vi "Operations.vi"(7 "References":T2, 8 "error in":errorcluster, 9 "BD":T1 items=["Server", "Local DB"], 10 "FilesPath":path, 11 "Queues in":T9) -> (0 "error out":errorcluster, 2 "Prop out":T12={"Raw Data"=[[0.0], [0.0234375], [0.9609375]], "Poperties"={"RMS values"=[], "Max"=[], "Min"=[], "A(8)"=[], "t"=0.0, "A(8) Axis"=0.0, "Aw"=[], "Ak 30min"=0.0, "Ak_axis"=0, "Spec"=[]}, "Power Spectrum / PSD"=[]}, 3 "Queues out":T9)   [LabVIEW 2019]
uses:
  Communication/TypeDef/#TypeDef_PropGraph.ctl
  Communication/TypeDef/#TypeDef_PropertiesToSave.ctl
  Queue/TypeDef/#TypeDef_App_Queues.ctl
  User Interface/TypeDef/#TypeDef_Enum_Buttons.ctl
  User Interface/TypeDef/#TypeDef_EventStructureConstant.ctl
  User Interface/TypeDef/#TypeDef_Enum_EventStructure.ctl
  Queue/TypeDef/#TypeDef_NetworkStream.ctl
  Communication/TypeDef/#TypeDef_FromMRtoPC.ctl
  Communication/TypeDef/#TypeDef_FromPCtoMR.ctl
  Communication/TypeDef/#TypeDef_Command.ctl
  Communication/TypeDef/#TypeDef_ErrorHandler_prop.ctl
  <vilib>/addons/database/Connection.llb/Conn ObjectReference.ctl
  Test/TypeDef/#TypeDef_DataToTest.ctl
  User Interface/TypeDef/#TypeDef_References.ctl
  User Interface/TypeDef/#TypeDef_Buttons.ctl
  User Interface/TypeDef/#TypeDef_ReferencesMeassurementProp.ctl
  User Interface/TypeDef/#TypeDef_ReferencesArchiveProp.ctl
  User Interface/TypeDef/#TypeDef_Lists.ctl
  User Interface/TypeDef/#TypeDef_MeasProp.ctl
  User Interface/TypeDef/#TypeDef_OpProp.ctl
  User Interface/TypeDef/#TypeDef_Enum_ModeOp.ctl
  DataBase/TypeDef/#TypeDef_DBMode.ctl
  DataBase/TypeDef/#TypeDef_FinalDataToDatabase.ctl
  Communication/TypeDef/#TypeDef_SetGet.ctl
  <vilib>/addons/database/NI_Database_API.lvlib
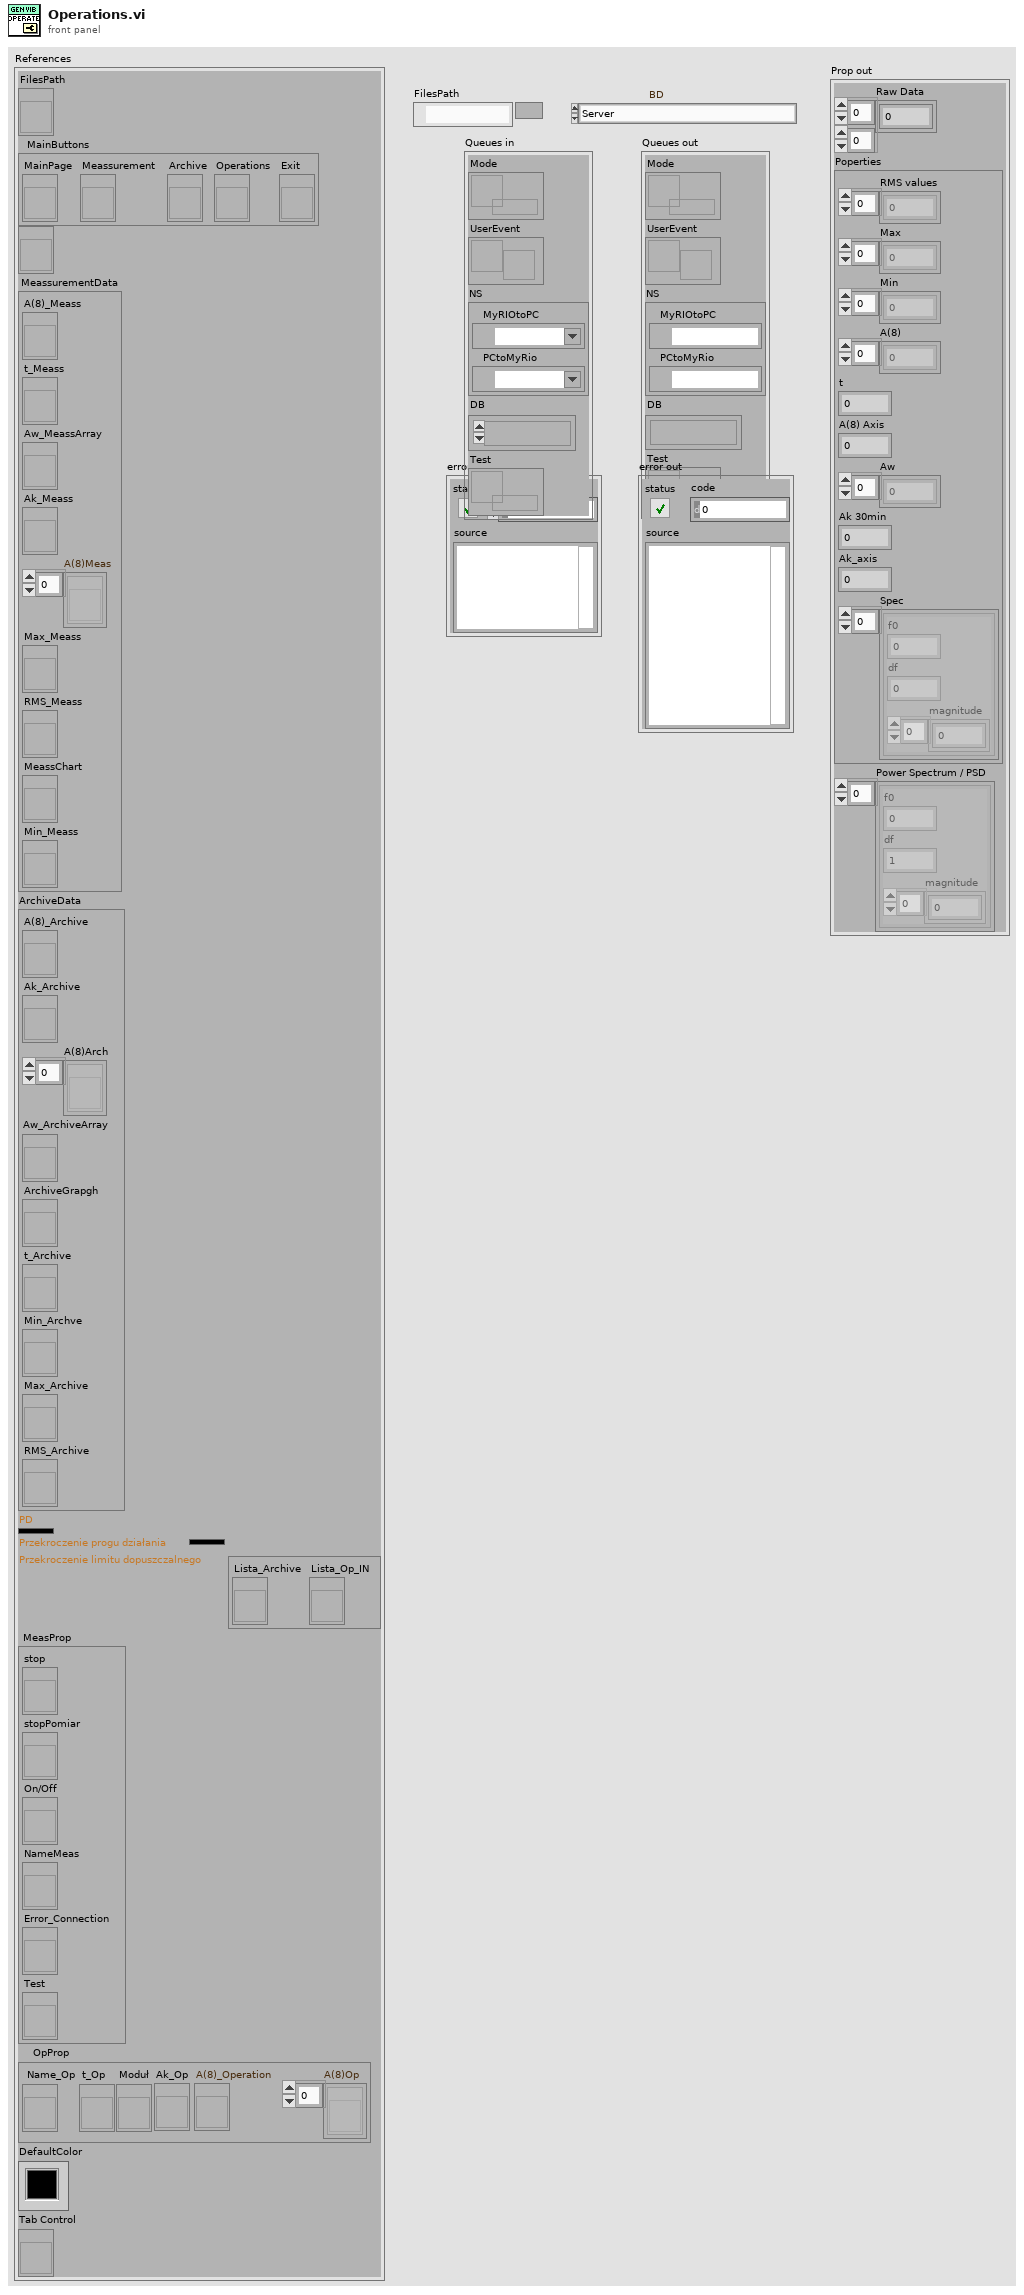
[diagram p1: front panel]
types:
  T1 = typedef "#TypeDef_DBMode.ctl" = u16
  T2 = typedef "#TypeDef_References.ctl" = cluster{"FilesPath":refnum<vi>, "MainButtons":T3, "Lista CTRL":refnum<vi>, "MeassurementData":T4, "ArchiveData":T5, "PD":u32, "LD":u32, "Lists":T6, "MeasProp":T7, "OpProp":T8, "DefaultColor":u32, "Tab Control":refnum<vi>}
  T3 = typedef "#TypeDef_Buttons.ctl" = cluster{"MainPage":refnum<vi>, "Meassurement":refnum<vi>, "Archive":refnum<vi>, "Operations":refnum<vi>, "Exit":refnum<vi>}
  T4 = typedef "#TypeDef_ReferencesMeassurementProp.ctl" = cluster{"A(8)_Meass":refnum<vi>, "t_Meass":refnum<vi>, "Aw_MeassArray":refnum<vi>, "Ak_Meass":refnum<vi>, "A(8)Meas":refnum<vi>[], "Max_Meass":refnum<vi>, "RMS_Meass":refnum<vi>, "MeassChart":refnum<vi>, "Min_Meass":refnum<vi>}
  T5 = typedef "#TypeDef_ReferencesArchiveProp.ctl" = cluster{"A(8)_Archive":refnum<vi>, "Ak_Archive":refnum<vi>, "A(8)Arch":refnum<vi>[], "Aw_ArchiveArray":refnum<vi>, "ArchiveGrapgh":refnum<vi>, "t_Archive":refnum<vi>, "Min_Archve":refnum<vi>, "Max_Archive":refnum<vi>, "RMS_Archive":refnum<vi>}
  T6 = typedef "#TypeDef_Lists.ctl" = cluster{"Lista_Archive":refnum<vi>, "Lista_Op_IN":refnum<vi>}
  T7 = typedef "#TypeDef_MeasProp.ctl" = cluster{"stop":refnum<vi>, "stopPomiar":refnum<vi>, "On/Off":refnum<vi>, "NameMeas":refnum<vi>, "Error_Connection":refnum<vi>, "Test":refnum<vi>}
  T8 = typedef "#TypeDef_OpProp.ctl" = cluster{"Name_Op":refnum<vi>, "t_Op":refnum<vi>, "Modu³":refnum<vi>, "Ak_Op":refnum<vi>, "A(8)_Operation":refnum<vi>, "A(8)Op":refnum<vi>[]}
  T9 = typedef "#TypeDef_App_Queues.ctl" = cluster{"Mode":refnum<queue>, "UserEvent":refnum<user-event>, "NS":T10, "DB":T11, "Test":refnum<queue>}
  T10 = typedef "#TypeDef_NetworkStream.ctl" = cluster{"MyRIOtoPC":refnum<k21>, "PCtoMyRio":refnum<k21>}
  T11 = typedef "NI_Database_API.lvlib/Conn ObjectReference.ctl" = refnum<k1>
  T12 = typedef "#TypeDef_PropGraph.ctl" = cluster{"Raw Data":dbl[][], "Poperties":T13, "Power Spectrum / PSD":cluster{"f0":dbl, "df":dbl, "magnitude":dbl[]}[]}
  T13 = typedef "#TypeDef_PropertiesToSave.ctl" = cluster{"RMS values":dbl[], "Max":dbl[], "Min":dbl[], "A(8)":dbl[], "t":dbl, "A(8) Axis":dbl, "Aw":dbl[], "Ak 30min":dbl, "Ak_axis":i32, "Spec":cluster{"f0":dbl, "df":dbl, "magnitude":dbl[]}[]}
  T14 = enum16{"open", "open or create", "create or replace", "create", "open (read-only)"}
  T15 = typedef "#TypeDef_SetGet.ctl" = enum16{"Set", "Get"}
  T16 = typedef "#TypeDef_FinalDataToDatabase.ctl" = cluster{"A8":dbl[], "Ak Aray":dbl[]}
  T17 = typedef "#TypeDef_Enum_ModeOp.ctl" = enum16{"Oblicz ekspozycjê dzienn¹", "Uœrednij"}
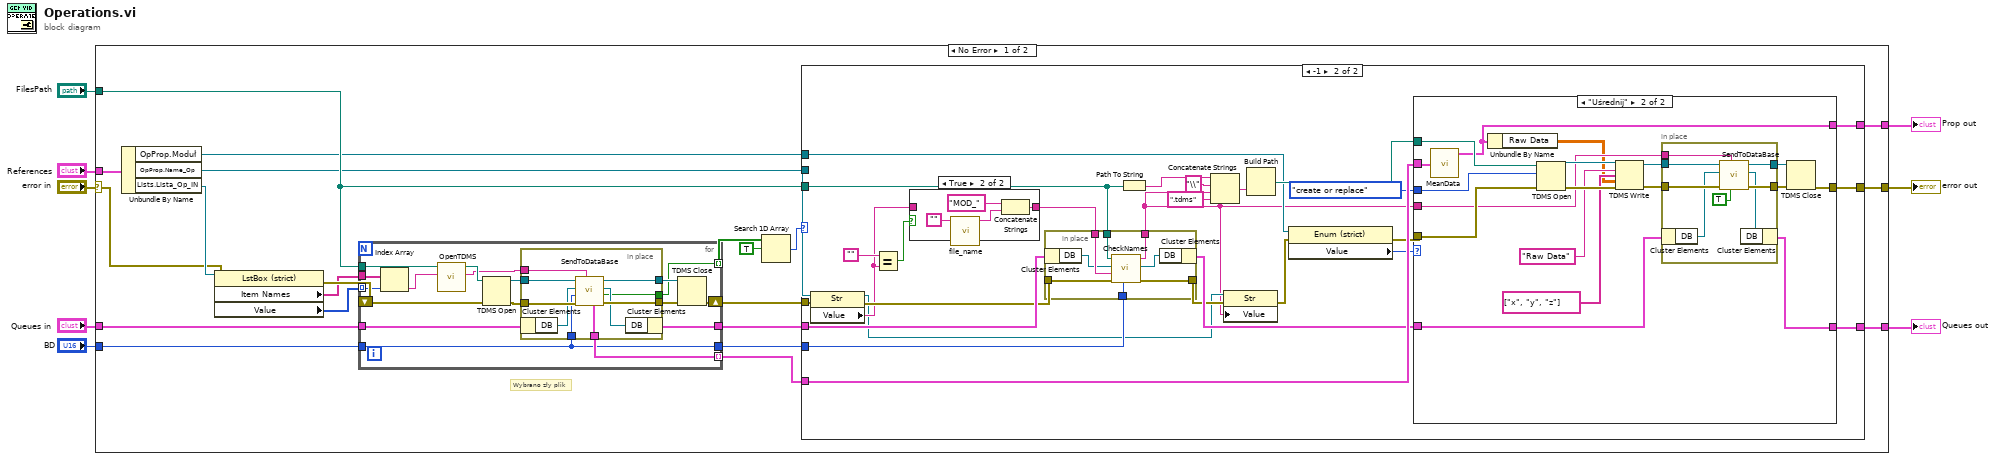
[diagram p0: block diagram]
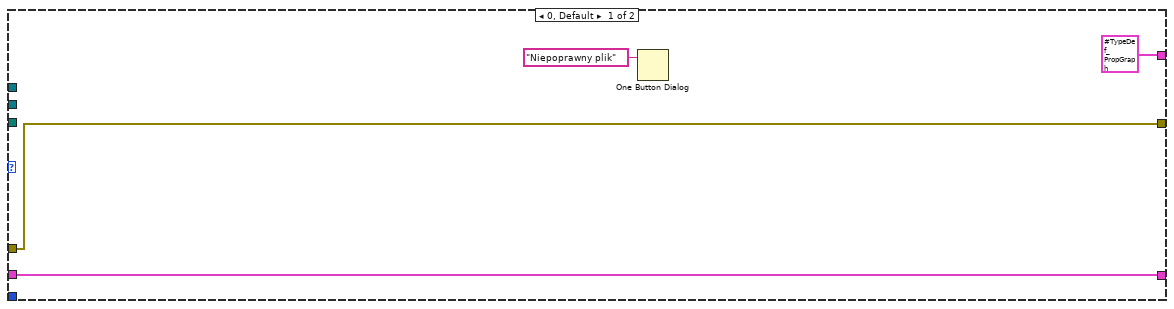
[diagram p2: hidden frame]
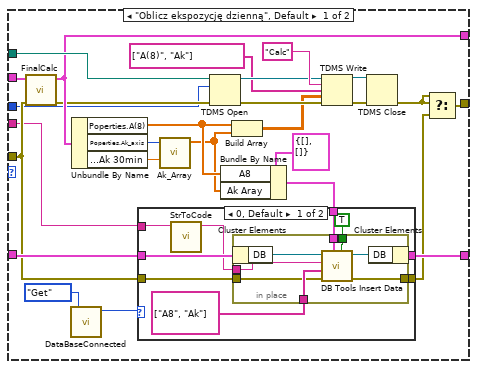
[diagram p4: hidden frame]
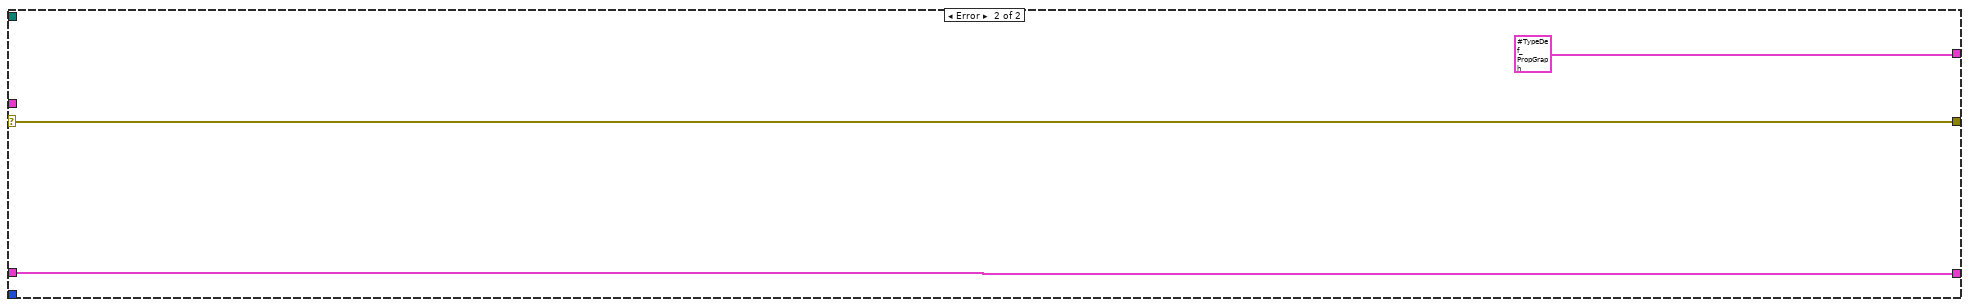
[diagram p6: hidden frame]
diagram:
  n1 = case shown="No Error" "error in" {
    selector: "error in" -> [w18 w174]
    tunnel: [w29 T12 {"Raw Data"=[[0.0], [0.0234375], [0.9609375]], "Poperties"={"RMS values"=[], "Max"=[], "Min"=[], "A(8)"=[], "t"=0.0, "A(8) Axis"=0.0, "Aw"=[], "Ak 30min"=0.0, "Ak_axis"=0, "Spec"=[]}, "Power Spectrum / PSD"=[]} ("Prop out")] -> w2
    tunnel: [w21 w175] -> w7
    tunnel: "Queues in" -> [w26 w175]
    tunnel: "References" -> [w24 _]
    tunnel: "FilesPath" -> [w22 _]
    tunnel: [w23 w174] -> w3
    tunnel: "BD" -> [w16 _]
    frame No Error {
      # "Wybrano z³y plik"
      n2 = Unbundle By Name(w24) -> ("OpProp.Modu³"=w17:refnum<vi>, "OpProp.Name_Op"=w12:refnum<vi>, "Lists.Lista_Op_IN"=w25:refnum<vi>)
      n3 = property class="LstBox (strict)"(reference=w25, error in=w18) -> (error out=w27:errorcluster, "Item Names"=w20:string[], "Value"=w19:i32[])  [unwired: 1 out]
      n4 = for {
        tunnel: w26 -> [w162]
        tunnel: [w161] -> w14
        shift-right: [w151] -> w13
        shift-left: w27 -> [w160]
        tunnel: w22 -> [w158]
        tunnel: [w154] -> w28 mode=indexing
        tunnel: w20 -> [w150]
        tunnel: w19 -> [w149] mode=indexing
        tunnel: w16 -> [w147]
        tunnel: [w147] -> w15
        tunnel: [w146] -> w10 mode=indexing
        n5 = Index Array(array=w150, index=w149) -> (element=w148:string)
        n6 = call "OpenTDMS.vi"("Name in"=w148, "FilesPath"=w158) -> ("Name out"=w155:string, "Path"=w157:path)  [unwired: 8 in]
        n7 = TDMS Open(8:w160, 11:w157) -> (0:w159:errorcluster, 3:w156:refnum<k34>)  [unwired: 5 in]
        n8 = in-place {
          in-place-border: [w172] -> w152
          in-place-border: [w171] -> w153
          in-place-border: w156 -> [w170]
          in-place-border: w159 -> [w169]
          in-place-border: w155 -> [w168]
          in-place-border: [w167] -> w154
          in-place-border: w147 -> [w164]
          in-place-border: [w163] -> w146
          n9 = in-place-cluster #1(w162) -> ("DB"=w166:T11)
          n10 = call "SendToDataBase.vi"("TableName"=w168, "error in"=w169, "BD_Op"=w164, "Connection in"=w166, "tdms file in"=w170) -> ("error out"=w171:errorcluster, "Modified?"=w163:bool, "Connection out"=w165:T11, "tdms file out"=w172:refnum<k34>, "PropGraph"=w167:T12)  [unwired: 2 in]
          n11 = in-place-cluster #1("DB"=w165) -> (w161:T9)
        }
        n12 = TDMS Close(8:w153, 11:w152) -> (0:w151:errorcluster)  [unwired: 1 out]
      }
      n13 = Search 1D Array(1D array=w10, element=TRUE) -> (index of element=w11:i32)  [unwired: 1 in]
      n14 = case shown="-1" w11 {
        tunnel: [T12 {"Raw Data"=[[0.0], [0.0234375], [0.9609375]], "Poperties"={"RMS values"=[], "Max"=[], "Min"=[], "A(8)"=[], "t"=0.0, "A(8) Axis"=0.0, "Aw"=[], "Ak 30min"=0.0, "Ak_axis"=0, "Spec"=[]}, "Power Spectrum / PSD"=[]} ("Poperties out") w61] -> w29
        tunnel: w28 -> [_ w60]
        tunnel: [w32 w55] -> w23
        tunnel: w22 -> [_ w54]
        tunnel: [w33 w52] -> w21
        tunnel: w17 -> [_ w49]
        tunnel: w15 -> [_ w47]
        tunnel: w14 -> [w33 w46]
        tunnel: w13 -> [w32 w44]
        tunnel: w12 -> [_ w42]
        frame 0, Default {
          n15 = One Button Dialog(message="Niepoprawny plik") -> ()  [unwired: 1 in, 1 out]
        }
        frame -1 {
          n16 = property class="Str"(reference=w42, error in=w44) -> (reference out=w37:refnum<vi>, error out=w43:errorcluster, "Value"=w39:string)
          n17 = Equal?(x="", y=w39) -> (x = y?=w40:bool)
          n18 = case shown="True" w40 {
            tunnel: [w62 w64] -> w53
            tunnel: w39 -> [w62 _]
            frame False {
            }
            frame True {
              n19 = call "file_name.vi"("String in"="") -> ("String out"=w66:string)  [unwired: 8 in]
              n20 = Concatenate Strings("MOD_" ("string"), w66) -> (w64:string)
            }
          }
          n21 = in-place {
            in-place-border: [w74] -> w36
            in-place-border: w43 -> [w73]
            in-place-border: w54 -> [w72]
            in-place-border: w53 -> [w71]
            in-place-border: [w70] -> w38
            in-place-border: w47 -> [w69]
            n22 = in-place-cluster #2(w46) -> ("DB"=w68:T11)
            n23 = call "CheckNames.vi"("BD"=w69, "error in"=w73, "Value in"=w71, "DB in"=w68, "Path"=w72) -> ("error out"=w70:errorcluster, "DB out"=w67:T11, "Value out"=w74:string)  [unwired: 4 in]
            n24 = in-place-cluster #2("DB"=w67) -> (w45:T9)
          }
          n25 = Path To String(path=w54) -> (string=w58:string)
          n26 = Concatenate Strings(w58, "\\" ("string"), w36, ".tdms" ("String in")) -> (w59:string)
          n27 = property class="Str"(reference=w37, error in=w38, "Value"=w36) -> (error out=w35:errorcluster)  [unwired: 1 out]
          n28 = Build Path(name or relative path=w59) -> (appended path=w56:path)  [unwired: 1 in]
          n29 = property class="Enum (strict)"(reference=w49, error in=w35) -> (error out=w51:errorcluster, "Value"=w50:T17)  [unwired: 1 out]
          n30 = case shown="\"Uœrednij\"" w50 {
            tunnel: w60 -> [w100 w137]
            tunnel: [w97 w124] -> w61
            tunnel: w56 -> [w99 w136]
            tunnel: w51 -> [w83 w134]
            tunnel: [w82 w125] -> w55
            tunnel: w36 -> [w77 w128]
            tunnel: w45 -> [w90 w122]
            tunnel: [w89 w121] -> w52
            tunnel: T14."create or replace" ("operation (0:open)") -> [w78 w120]
            frame "Oblicz ekspozycjê dzienn¹", Default {
              n31 = call "FinalCalc.vi"("Prop"=w100) -> ("Prop out"=w97:T12)  [unwired: 10 in]
              n32 = call "DataBaseConnected.vi"("Get/Set"=#TypeDef_SetGet."Get") -> ("BD out"=w75:T1)  [unwired: 10 in]
              n33 = Unbundle By Name(w97) -> ("Poperties.A(8)"=w85:dbl[], "Poperties.Ak_axis"=w88:i32, "Poperties.Ak 30min"=w87:dbl)
              n34 = call "Ak_Array.vi"("Ak 30min"=w87, "Ak_axis"=w88) -> ("Ak Aray"=w84:dbl[])  [unwired: 9 in]
              n35 = TDMS Open(8:w83, 10:w78, 11:w99) -> (0:w98:errorcluster, 3:w93:refnum<k34>)  [unwired: 4 in]
              n36 = Bundle By Name(cluster=T16 {"A8"=[], "Ak Aray"=[]}, "A8"=w85, "Ak Aray"=w84) -> (w79:T16)
              n37 = case shown="0, Default" w75 {
                tunnel: w90 -> [w109 w118]
                tunnel: [w108 w118] -> w89
                tunnel: w83 -> [w106 w119]
                tunnel: [w105 w119] -> w81
                tunnel: w79 -> [w104 _]
                tunnel: w77 -> [w102 _]
                frame 0, Default {
                  n38 = call "StrToCode.vi"("Name in"=w102) -> ("Name out"=w101:string)  [unwired: 10 in]
                  n39 = in-place {
                    in-place-border: string[] ["A8", "Ak"] ("columns") -> [w115]
                    in-place-border: w106 -> [w114]
                    in-place-border: [w113] -> w105
                    in-place-border: w104 -> [w112]
                    in-place-border: TRUE -> [w111]
                    in-place-border: w101 -> [w110]
                    n40 = in-place-cluster #3(w109) -> ("DB"=w117:T11)
                    n41 = call <vilib>:"DB Tools Insert Data.vi"("create table? (F)"=w111, "data"=w112, "error in (no error)"=w114, "columns"=w115, "table"=w110, "connection reference"=w117) -> ("error out"=w113:errorcluster, "connection reference out"=w116:T11)  [unwired: 4 in]
                    n42 = in-place-cluster #3("DB"=w116) -> (w108:T9)
                  }
                }
                frame 1 {
                }
              }
              n43 = Build Array(w85, w84) -> (w91:dbl[][])
              n44 = TDMS Write(0:w93, 5:"Calc" ("group name in (Untitled)"), 7:string[] ["A(8)", "Ak"] ("channel name(s) in (Untitled)"), 9:w91, 11:w98) -> (4:w95:refnum<k34>, 15:w96:errorcluster)  [unwired: 1 in, 2 out]
              n45 = TDMS Close(8:w96, 11:w95) -> (0:w80:errorcluster)  [unwired: 1 out]
              n46 = Select(t=w80, s=w80, f=w81) -> (s? t:f=w82:errorcluster)
            }
            frame "Uœrednij" {
              n47 = call "MeanData.vi"("Prop in"=w137) -> ("Poperties out"=w124:T12)  [unwired: 10 in]
              n48 = Unbundle By Name(w124) -> ("Raw Data"=w123:dbl[][])
              n49 = TDMS Open(8:w134, 10:w120, 11:w136) -> (0:w133:errorcluster, 3:w135:refnum<k34>)  [unwired: 4 in]
              n50 = TDMS Write(0:w135, 5:"Raw Data" ("group name in (Untitled)"), 7:string[] ["x", "y", "z"] ("channel name(s) in (Untitled)"), 9:w123, 11:w133) -> (4:w130:refnum<k34>, 15:w129:errorcluster)  [unwired: 1 in, 2 out]
              n51 = in-place {
                in-place-border: w130 -> [w145]
                in-place-border: w129 -> [w144]
                in-place-border: w128 -> [w143]
                in-place-border: [w141] -> w127
                in-place-border: [w140] -> w126
                n52 = in-place-cluster #4(w122) -> ("DB"=w139:T11)
                n53 = call "SendToDataBase.vi"("Put in?"=TRUE, "TableName"=w143, "error in"=w144, "Connection in"=w139, "tdms file in"=w145) -> ("error out"=w141:errorcluster, "Connection out"=w138:T11, "tdms file out"=w140:refnum<k34>)  [unwired: 2 in, 2 out]
                n54 = in-place-cluster #4("DB"=w138) -> (w121:T9)
              }
              n55 = TDMS Close(8:w127, 11:w126) -> (0:w125:errorcluster)  [unwired: 1 out]
            }
          }
        }
      }
    }
    frame Error {
    }
  }
  "Prop out" <- w2
  "Queues out" <- w7
  "error out" <- w3
